vi "_DServerReplyToExecuteCommand.vi"(1 "argio":cluster{"num data":u8[], "str data":string[]}, 2 "client request":T1={"Request Id"=0, "Source Id"=0, "Request Type"=enum."UNKNOWN_REQUEST", "Device Class Name"="unspecified/device/name", "Device Name"="unspecified_cmd_or_attr_name", "Cmd or Attr Name"="unspecified_cmd_or_attr_name", "Client Request Data"={"write attribute value"={"dimx"=0, "dimy"=0, "data"=[], "data_type"=enum."UNKNOWN_DATA_TYPE"}, "exec. command argin"={"num data"=[], "str data"=[]}}}, 3 "error in":errorcluster) -> (0 "error out":errorcluster)   [LabVIEW 2014, in "tango.lvlib"]
uses:
  tango.lvlib
  Client Request Handling/Typedefs/_DServerClientRequest.ctl
  Client Request Handling/Typedefs/_DServerClientRequestType.ctl
  Client Request Handling/Typedefs/_DServerClientRequestData.ctl
  Client Request Handling/Typedefs/_GenericDataBuffer.ctl
  Common VIs/Typedefs/_AttributeDataType_t.ctl
  vis/tango_binding.so
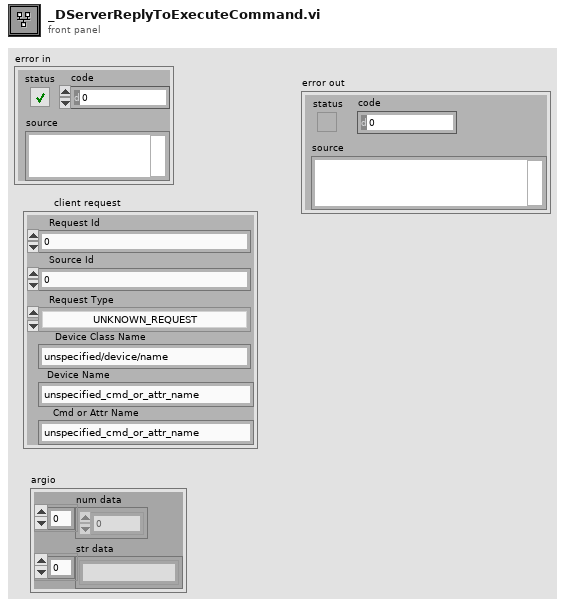
[diagram p1: front panel]
types:
  T1 = typedef "tango.lvlib/_DServerClientRequest.ctl" = cluster{"Request Id":u32, "Source Id":u32, "Request Type":T2, "Device Class Name":string, "Device Name":string, "Cmd or Attr Name":string, "Client Request Data":T3}
  T2 = typedef "tango.lvlib/_DServerClientRequestType.ctl" = enum16{"EXEC_CMD", "READ_ATTR", "WRITE_ATTR", "UNKNOWN_REQUEST"}
  T3 = typedef "tango.lvlib/_DServerClientRequestData.ctl" = cluster{"write attribute value":T4, "exec. command argin":cluster{"num data":u8[], "str data":string[]}}
  T4 = typedef "tango.lvlib/_GenericDataBuffer.ctl" = cluster{"dimx":u32, "dimy":u32, "data":u8[], "data_type":T5}
  T5 = typedef "tango.lvlib/_AttributeDataType_t.ctl" = enum16{"STATE_SCA", "STATE_SPE", "STATE_IMG", "STRING_SCA", "STRING_SPE", "STRING_IMG", "BOOL_SCA", "BOOL_SPE", "BOOL_IMG", "UCHAR_SCA", "UCHAR_SPE", "UCHAR_IMG", "SHORT_SCA", "SHORT_SPE", "SHORT_IMG", "USHORT_SCA", "USHORT_SPE", "USHORT_IMG", "LONG_SCA", "LONG_SPE", "LONG_IMG", "ULONG_SCA", "ULONG_SPE", "ULONG_IMG", "LONG64_SCA", "LONG64_SPE", "LONG64_IMG", "ULONG64_SCA", "ULONG64_SPE", "ULONG64_IMG", "FLOAT_SCA", "FLOAT_SPE", "FLOAT_IMG", "DOUBLE_SCA", "DOUBLE_SPE", "DOUBLE_IMG", "ENUM_SCA", "UNKNOWN_DATA_TYPE"}
  T6 = cluster{"Request Id":u32, "Source Id":u32, u32, "error stack":string[]}
  T7 = cluster{cluster{"Request Id":u32, "Source Id":u32, u32, "error stack":string[]}, "argio":cluster{"num data":u8[], "str data":string[]}}
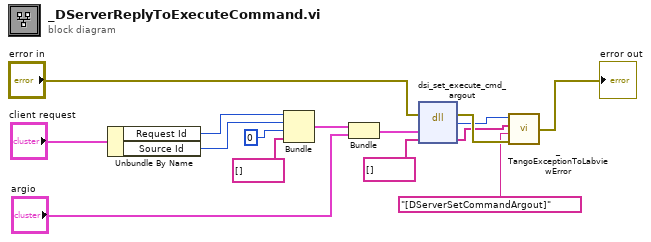
[diagram p0: block diagram]
diagram:
  n1 = Unbundle By Name("client request") -> ("Request Id"=w7:u32, "Source Id"=w6:u32)
  n2 = Bundle("Request Id"=w7, "Source Id"=w6, u32 0, "error stack"=string[] []) -> (w3:T6)  [unwired: 1 in]
  n3 = Bundle(w3, "argio"="argio") -> (w2:T7)  [unwired: 1 in]
  n4 = dll-call lib="home/nicolas/bindings/labview-binding@github.tango-controls/vis/tango_binding.*" fn="dsi_set_execute_cmd_argout"(error in="error in", "attribute_value"=w2, "error_stack"=string[] [] ("error stack")) -> (error out=w12:errorcluster, "return type"=w10:i32, "error_stack"=w11:string[])  [unwired: 3 in, 1 out]
  n5 = call "_TangoExceptionToLabviewError.vi"("error in"=w12, "location"="[DServerSetCommandArgout]", "error stack"=w11, "error code"=w10) -> ("error out"=→"error out":errorcluster)
